vi "FPGA.vi"   [LabVIEW 2016]
uses:
  <vilib>/rvi/interface/nirviReadWriteControl/nirviReadWriteControl.xnode
  Globale Variable/Globale Variable.vi
  <vilib>/rvi/interface/nirviOpenFPGA/nirviOpenFPGA.xnode
  <vilib>/rvi/interface/nirviMethod/nirviMethod.xnode
  <vilib>/FPGAPlugInAG/Dynamic/niLvFpga_Run_Dynamic.vi
  cRIO SUPERFINAL 2.6/FPGA Bitfiles/SUPERFINAL2.7_FPGATarget_CountingFPGA_xv91Jg-Kp9s.lvbitx
  <vilib>/FPGAPlugInAG/cRIO-9067/niLvFpga_Open_cRIO-9067.vi
  <vilib>/rvi/interface/common/dynamic/niFpgaDynamicAddResources.vi
  NiFpgaLv.dll
  <vilib>/Utility/error.llb/Error Cluster From Error Code.vi
  <vilib>/rvi/interface/Simulation/niFpgaSimulationCallBeginRW.vi
  <vilib>/rvi/errors/niLvFpgaAdjustHostInterfaceError.vi
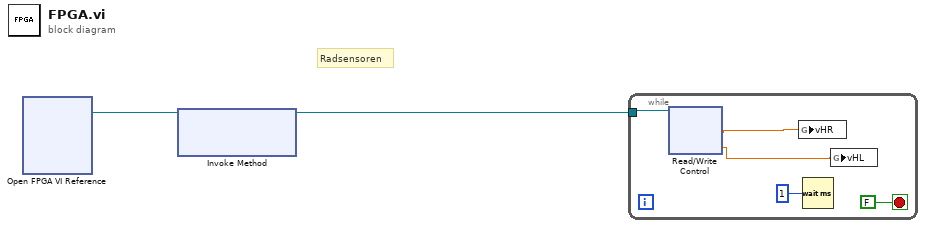
[diagram p0: block diagram]
diagram:
  # "Radsensoren"
  n1 = xnode "Open FPGA VI Reference"() -> ("FPGA VI Reference Out"=w1:refnum<k20>)  [unwired: 2 in, 1 out]
  n2 = xnode "Invoke Method"("FPGA VI Reference In"=w1) -> ("FPGA VI Reference Out"=w2:refnum<k20>)  [unwired: 2 in, 1 out]
  n3 = while {
    tunnel: w2 -> [w7]
    stop <- FALSE stop-if-true
    n4 = xnode "Read/Write Control"("FPGA VI Reference In"=w7) -> ("vHR"=w4:sgl, "vHL"=w3:sgl)  [unwired: 1 in, 2 out]
    n5 = global write "Globale Variable.vi" "vHR"(w4) -> ()
    n6 = Wait (ms)(milliseconds to wait=u32 1) -> ()  [unwired: 1 out]
    n7 = global write "Globale Variable.vi" "vHL"(w3) -> ()
  }
